vi "JSON RPC Server.vi"   [LabVIEW 2013]
uses:
  <vilib>/addons/zeromq/socket_type.ctl
  JSON RPC Request.ctl
  JSON RPC Response.ctl
  <vilib>/addons/zeromq/zmq_context.lvclass
  <vilib>/addons/zeromq/zeromq.lvlib
  <vilib>/addons/zeromq/zmq_socket.lvclass
types:
  T1 = typedef "zeromq.lvlib/socket_type.ctl" = enum8{"ZMQ_PAIR", "ZMQ_PUB", "ZMQ_SUB", "ZMQ_REQ", "ZMQ_REP", "ZMQ_DEALER", "ZMQ_ROUTER", "ZMQ_PULL", "ZMQ_PUSH", "ZMQ_XPUB", "ZMQ_XSUB"}
  T2 = typedef "JSON RPC Request.ctl" = cluster{"id":dbl, "method":string, "jsonrpc":string, "params":string}
  T3 = typedef "JSON RPC Response.ctl" = cluster{"id":dbl, "result":string, "jsonrpc":string}
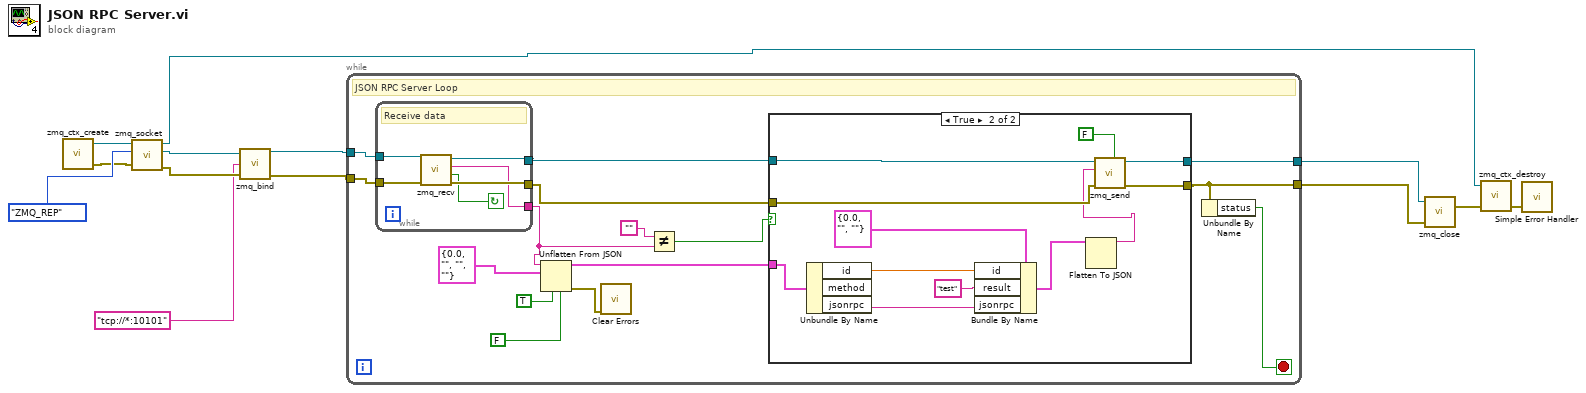
[diagram p0: block diagram]
diagram:
  n1 = call <vilib>:"zmq_ctx_create.vi"() -> ("error out"=w12:errorcluster, "context out"=w8:refnum<class "zmq_context.lvclass">)  [unwired: 4 in]
  n2 = call <vilib>:"zmq_socket.vi"("error in"=w12, "socket type"=socket_type."ZMQ_REP", "context in"=w8) -> ("error out"=w11:errorcluster, "socket out"=w10:refnum<class "zmq_socket.lvclass">, "context out"=w1:refnum<class "zmq_context.lvclass">)  [unwired: 2 in]
  n3 = call <vilib>:"zmq_bind.vi"("error in"=w11, "endpoint"="tcp://*:10101", "socket in"=w10) -> ("error out"=w6:errorcluster, "socket out"=w7:refnum<class "zmq_socket.lvclass">)  [unwired: 1 in]
  n4 = while {
    tunnel: [w17] -> w3
    tunnel: w7 -> [w27]
    tunnel: w6 -> [w26]
    tunnel: [w16] -> w2
    stop <- w24 stop-if-true
    # "JSON RPC Server Loop"
    n5 = while {
      tunnel: [w48] -> w25
      tunnel: [w47] -> w28
      tunnel: w27 -> [w45]
      tunnel: w26 -> [w44]
      tunnel: [w43] -> w20
      stop <- w46 continue-if-true
      # "Receive data"
      n6 = call <vilib>:"zmq_recv.vi"("error in"=w44, "socket in"=w45) -> ("error out"=w48:errorcluster, "more?"=w46:bool, "data"=w43:string, "socket out"=w47:refnum<class "zmq_socket.lvclass">)  [unwired: 3 in, 1 out]
    }
    n7 = Unflatten From JSON(JSON string=w20, type and defaults=T2 {"id"=0.0, "method"="", "jsonrpc"="", "params"=""} ("JSON RPC Request"), default null elements? (F)=TRUE, strict validation? (F)=FALSE) -> (value=w22:T2, error out=w14:errorcluster)  [unwired: 3 in]
    n8 = call <vilib>:"Clear Errors.vi"("error in (no error)"=w14) -> ()  [unwired: 6 in, 1 out]
    n9 = Not Equal?(x="", y=w20) -> (x != y?=w18:bool)
    n10 = case shown="True" w18 {
      tunnel: w28 -> [w29 w42]
      tunnel: w25 -> [w30 w41]
      tunnel: w22 -> [_ w40]
      tunnel: [w30 w32] -> w17
      tunnel: [w29 w31] -> w16
      frame False {
      }
      frame True {
        n11 = Unbundle By Name(w40) -> ("id"=w35:dbl, "jsonrpc"=w36:string)  [unwired: 1 out]
        n12 = Bundle By Name(cluster=T3 {"id"=0.0, "result"="", "jsonrpc"=""} ("JSON RPC Response"), "id"=w35, "result"="test", "jsonrpc"=w36) -> (w37:T3)
        n13 = Flatten To JSON(anything=w37) -> (JSON string=w33:string)  [unwired: 2 in, 1 out]
        n14 = call <vilib>:"zmq_send.vi"("error in"=w41, "data"=w33, "socket in"=w42, "more? (F)"=FALSE) -> ("error out"=w32:errorcluster, "socket out"=w31:refnum<class "zmq_socket.lvclass">)  [unwired: 3 in]
      }
    }
    n15 = Unbundle By Name(w17) -> ("status"=w24:bool)
  }
  n16 = call <vilib>:"zmq_close.vi"("error in"=w3, "socket"=w2) -> ("error out"=w5:errorcluster)  [unwired: 3 in]
  n17 = call <vilib>:"zmq_ctx_destroy.vi"("error in"=w5, "context in"=w1) -> ("error out"=w4:errorcluster)  [unwired: 3 in]
  n18 = call <vilib>:"Simple Error Handler.vi"("error in (no error)"=w4) -> ()  [unwired: 4 in, 5 out]
